vi "Analyse.vi"(8 "error in (no error)":errorcluster, 10 "ImageData":T1, 11 "AbsorptionDS in":refnum<class "Absorption2.lvclass">) -> (0 "error out":errorcluster, 3 "AbsorptionDS out":refnum<class "Absorption2.lvclass">)   [LabVIEW 2011, in "Tools.lvlib" / "Imaging.lvlib" / "Absorption2.lvclass"]
uses:
  Absorption2.lvclass
  Absorption2.lvclass/Absorption2.ctl
  AbsorptionAnalyser/AbsorptionAnalyser.lvclass
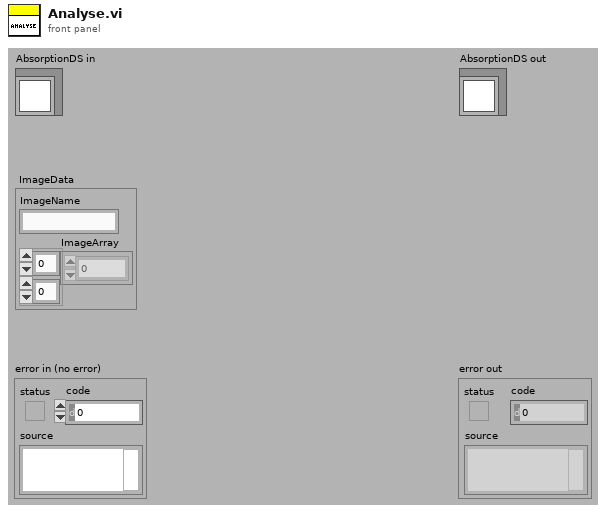
[diagram p1: front panel]
types:
  T1 = cluster{"ImageName":string, "ImageArray":sgl[][]}
  T2 = cluster{"ImageName":string, "ImageArray":sgl[][]}[]
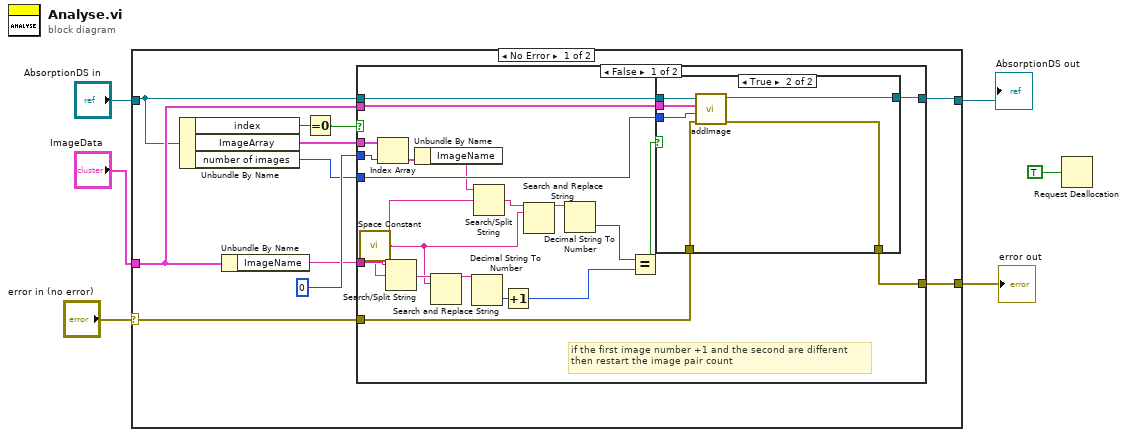
[diagram p0: block diagram]
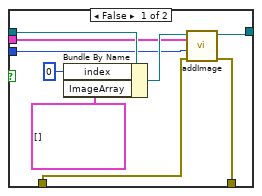
[diagram p2: hidden frame]
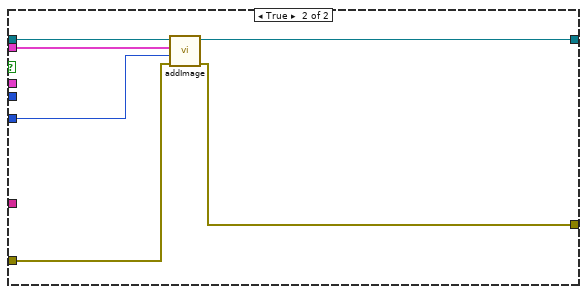
[diagram p3: hidden frame]
diagram:
  n1 = case shown="No Error" "error in (no error)" {
    selector: "error in (no error)" -> [w16 w59]
    tunnel: [w15 w59] -> w3
    tunnel: [w17 w60] -> w2
    tunnel: "AbsorptionDS in" -> [w7 w60]
    tunnel: "ImageData" -> [w14 _]
    frame No Error {
      n2 = Unbundle By Name(w7) -> ("index"=w10:i32, "ImageArray"=w13:T2, "number of images"=w8:i32)
      n3 = Unbundle By Name(w14) -> ("ImageName"=w9:string)
      n4 = Equal To 0?(x=w10) -> (x = 0?=w11:bool)
      n5 = case shown="False" w11 {
        tunnel: [w32 w58] -> w17
        tunnel: w16 -> [w30 w57]
        tunnel: [w29 w56] -> w15
        tunnel: w14 -> [w31 w55]
        tunnel: w7 -> [w33 w54]
        tunnel: w13 -> [w36 _]
        tunnel: 0 -> [w37 _]
        tunnel: w9 -> [w27 _]
        tunnel: w8 -> [w28 w53]
        frame False {
          # "if the first image number +1 and the second are different\nthen restart the image pair count"
          n6 = call <vilib>:"Space Constant.vi"() -> ("String"=w20:string)
          n7 = Index Array(array=w36, index=w37) -> (element=w35:T1)
          n8 = Search/Split String(string=w27, search string/char (-)=w20) -> (match + rest of string=w25:string)  [unwired: 1 in, 2 out]
          n9 = Unbundle By Name(w35) -> ("ImageName"=w26:string)
          n10 = Search and Replace String(input string=w25, search string=w20) -> (result string=w24:string)  [unwired: 6 in, 3 out]
          n11 = Decimal String To Number(string=w24) -> (number=w23:i32)  [unwired: 2 in, 1 out]
          n12 = Search/Split String(string=w26, search string/char (-)=w20) -> (match + rest of string=w21:string)  [unwired: 1 in, 2 out]
          n13 = Increment(x=w23) -> (x+1=w18:i32)
          n14 = Search and Replace String(input string=w21, search string=w20) -> (result string=w22:string)  [unwired: 6 in, 3 out]
          n15 = Decimal String To Number(string=w22) -> (number=w19:i32)  [unwired: 2 in, 1 out]
          n16 = Equal?(x=w19, y=w18) -> (x = y?=w34:bool)
          n17 = case shown="True" w34 {
            tunnel: w33 -> [w45 w52]
            tunnel: [w43 w51] -> w32
            tunnel: w31 -> [w41 w50]
            tunnel: w30 -> [w40 w49]
            tunnel: [w39 w48] -> w29
            tunnel: w28 -> [w38 w47]
            frame False {
              n18 = Bundle By Name(cluster=w45, "index"=0, "ImageArray"=T2 []) -> (w44:refnum<class "Absorption2.lvclass">)
              n19 = call "addImage.vi"("error in (no error)"=w40, "number of images"=w38, "ImageData"=w41, "AbsorptionAnalyser in"=w44) -> ("error out"=w39:errorcluster, "AbsorptionAnalyser out"=w43:refnum<class "Absorption2.lvclass">)  [unwired: 6 in]
            }
            frame True {
              n20 = call "addImage.vi"("error in (no error)"=w49, "number of images"=w47, "ImageData"=w50, "AbsorptionAnalyser in"=w52) -> ("error out"=w48:errorcluster, "AbsorptionAnalyser out"=w51:refnum<class "Absorption2.lvclass">)  [unwired: 6 in]
            }
          }
        }
        frame True {
          n21 = call "addImage.vi"("error in (no error)"=w57, "number of images"=w53, "ImageData"=w55, "AbsorptionAnalyser in"=w54) -> ("error out"=w56:errorcluster, "AbsorptionAnalyser out"=w58:refnum<class "Absorption2.lvclass">)  [unwired: 6 in]
        }
      }
    }
    frame Error {
    }
  }
  "error out" <- w3
  "AbsorptionDS out" <- w2
  n22 = Request Deallocation(TRUE ("flag")) -> ()
